vi "Keyence Handler_EP.vi"(8 "error in (no error)":errorcluster, 11 "Message Queues out":T5) -> (0 "error out":errorcluster, 3 "Message Queue":refnum<queue>)   [LabVIEW 2014]
uses:
  support/Message Queue/Message Queue.lvlib
  support/Message Queue/Lossy Enqueue Message (Single).vi
  <vilib>/ErrorRing/Error Ring.xnode
  <vilib>/ethernetip/ethernetip.lvlib
  <vilib>/Utility/error.llb/Error Cluster From Error Code.vi
  <vilib>/ethernetip/ethernetip.llb/ethernetip.ctl
  JXC Data Cluster_EP.ctl
  Control_EP.ctl
  Status_EP.ctl
  support/Message Queue/Message Cluster.ctl
  support/Message Queue/All Message Queues.ctl
panel:
  out "JXC Data Cluster":T1={"State Text"="", "Communication Opened"=FALSE, "Ethernet IP Session"="", "Status"={"BUSY"=FALSE, "SVRE"=FALSE, "SETON"=FALSE, "INP"=FALSE, "ESTOP"=FALSE, "ALARM"=FALSE, "READY"=FALSE, "Current Position"=0, "Current Position mm"=0.0, "Current Speed"=0, "Current Pushing Force"=0, "Target Position"=0, "Target Position mm"=0.0, "Alarm"=0, "Record number"=0}, "Control"={"Record number"=0, "HOLD"=FALSE, "SVON"=FALSE, "DRIVE"=FALSE, "RESET"=FALSE, "SETUP"=FALSE, "JOG-"=FALSE, "JOG+"=FALSE, "FLGTH"=FALSE}, "network path"="192.168.1.250"}
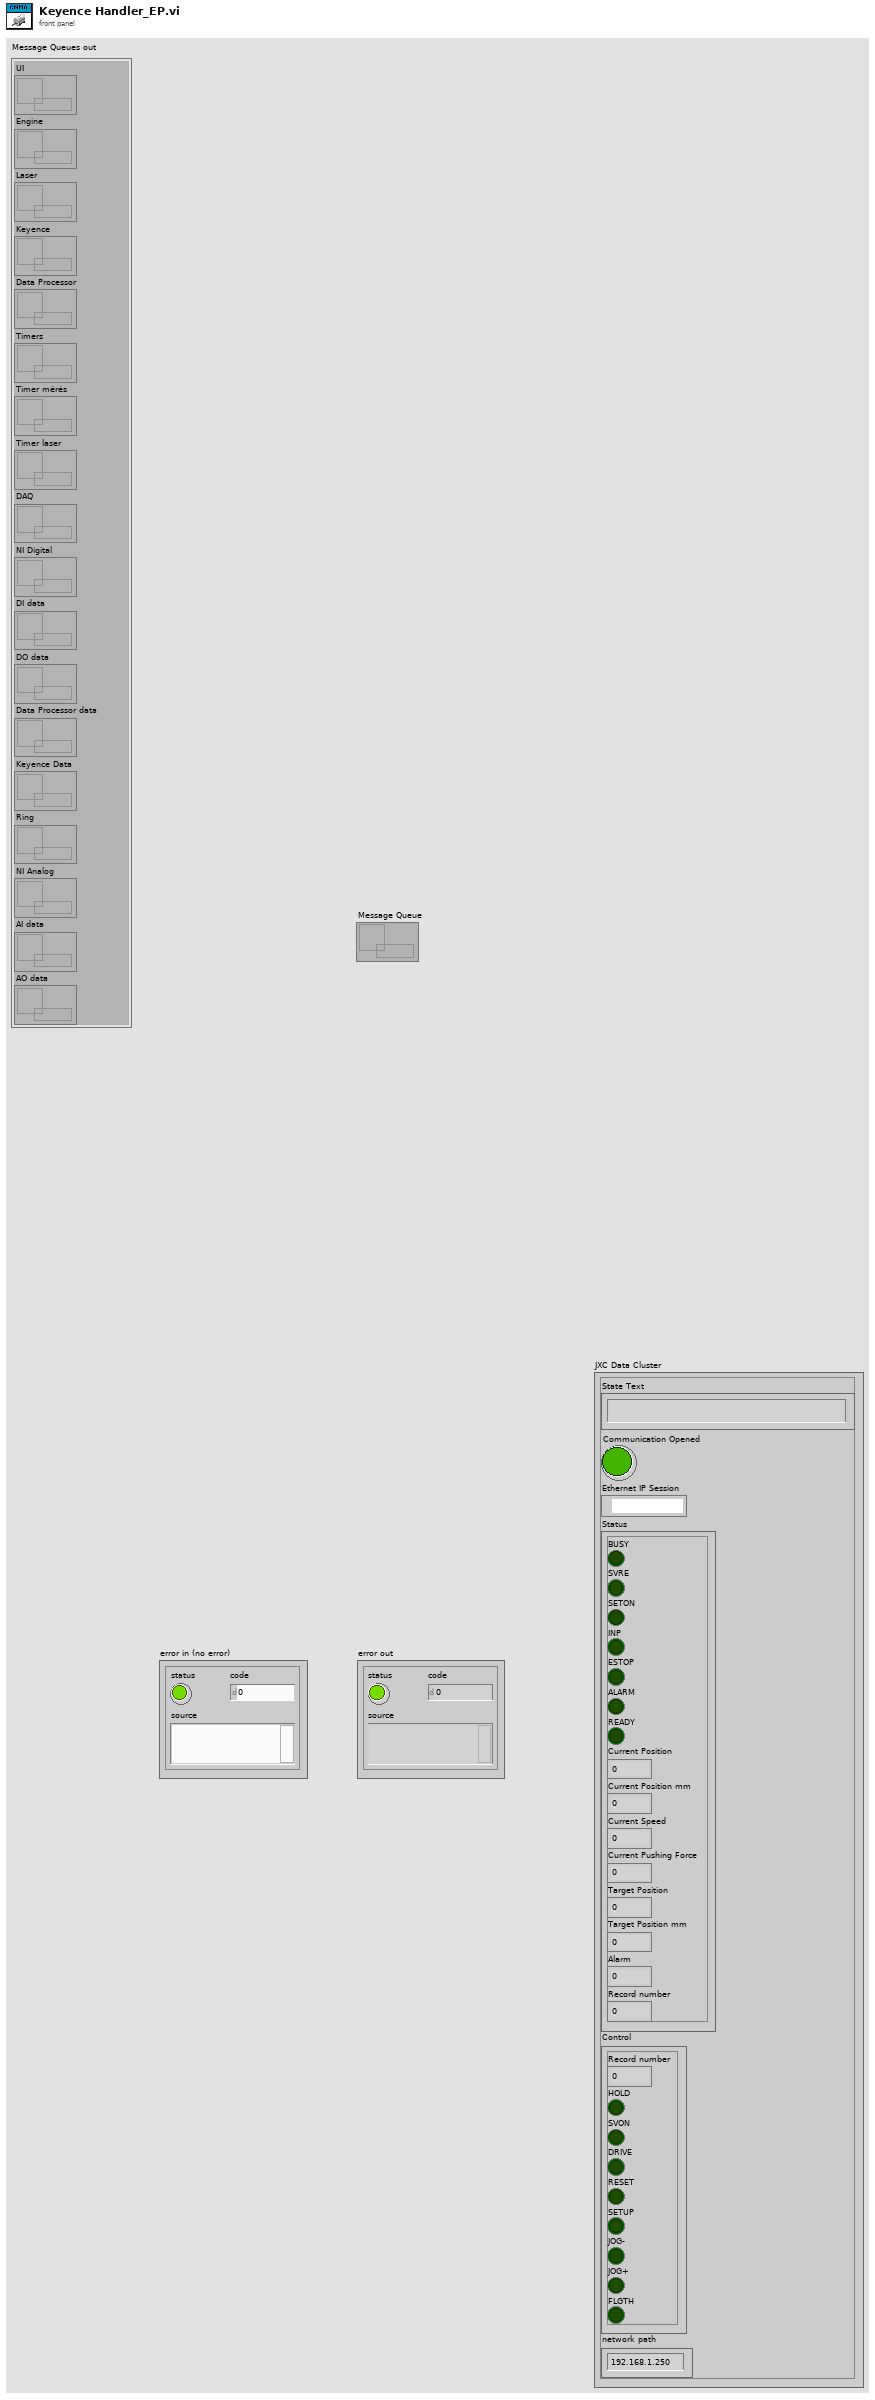
[diagram p1: front panel]
types:
  T1 = typedef "JXC Data Cluster_EP.ctl" = cluster{"State Text":string, "Communication Opened":bool, "Ethernet IP Session":T2, "Status":T3, "Control":T4, "network path":string}
  T2 = typedef "ethernetip.lvlib/ethernetip.ctl" = refnum<k21>
  T3 = typedef "Status_EP.ctl" = cluster{"BUSY":bool, "SVRE":bool, "SETON":bool, "INP":bool, "ESTOP":bool, "ALARM":bool, "READY":bool, "Current Position":u32, "Current Position mm":dbl, "Current Speed":u16, "Current Pushing Force":u16, "Target Position":u32, "Target Position mm":dbl, "Alarm":u8, "Record number":u32}
  T4 = typedef "Control_EP.ctl" = cluster{"Record number":u32, "HOLD":bool, "SVON":bool, "DRIVE":bool, "RESET":bool, "SETUP":bool, "JOG-":bool, "JOG+":bool, "FLGTH":bool}
  T5 = typedef "Message Queue.lvlib/All Message Queues.ctl" = cluster{"UI":refnum<queue>, "Engine":refnum<queue>, "Laser":refnum<queue>, "Keyence":refnum<queue>, "Data Processor":refnum<queue>, "Timers":refnum<queue>, "Timer mérés":refnum<queue>, "Timer laser":refnum<queue>, "DAQ":refnum<queue>, "NI Digital":refnum<queue>, "DI data":refnum<queue>, "DO data":refnum<queue>, "Data Processor data":refnum<queue>, "Keyence Data":refnum<queue>, "Ring":refnum<queue>, "NI Analog":refnum<queue>, "AI data":refnum<queue>, "AO data":refnum<queue>}
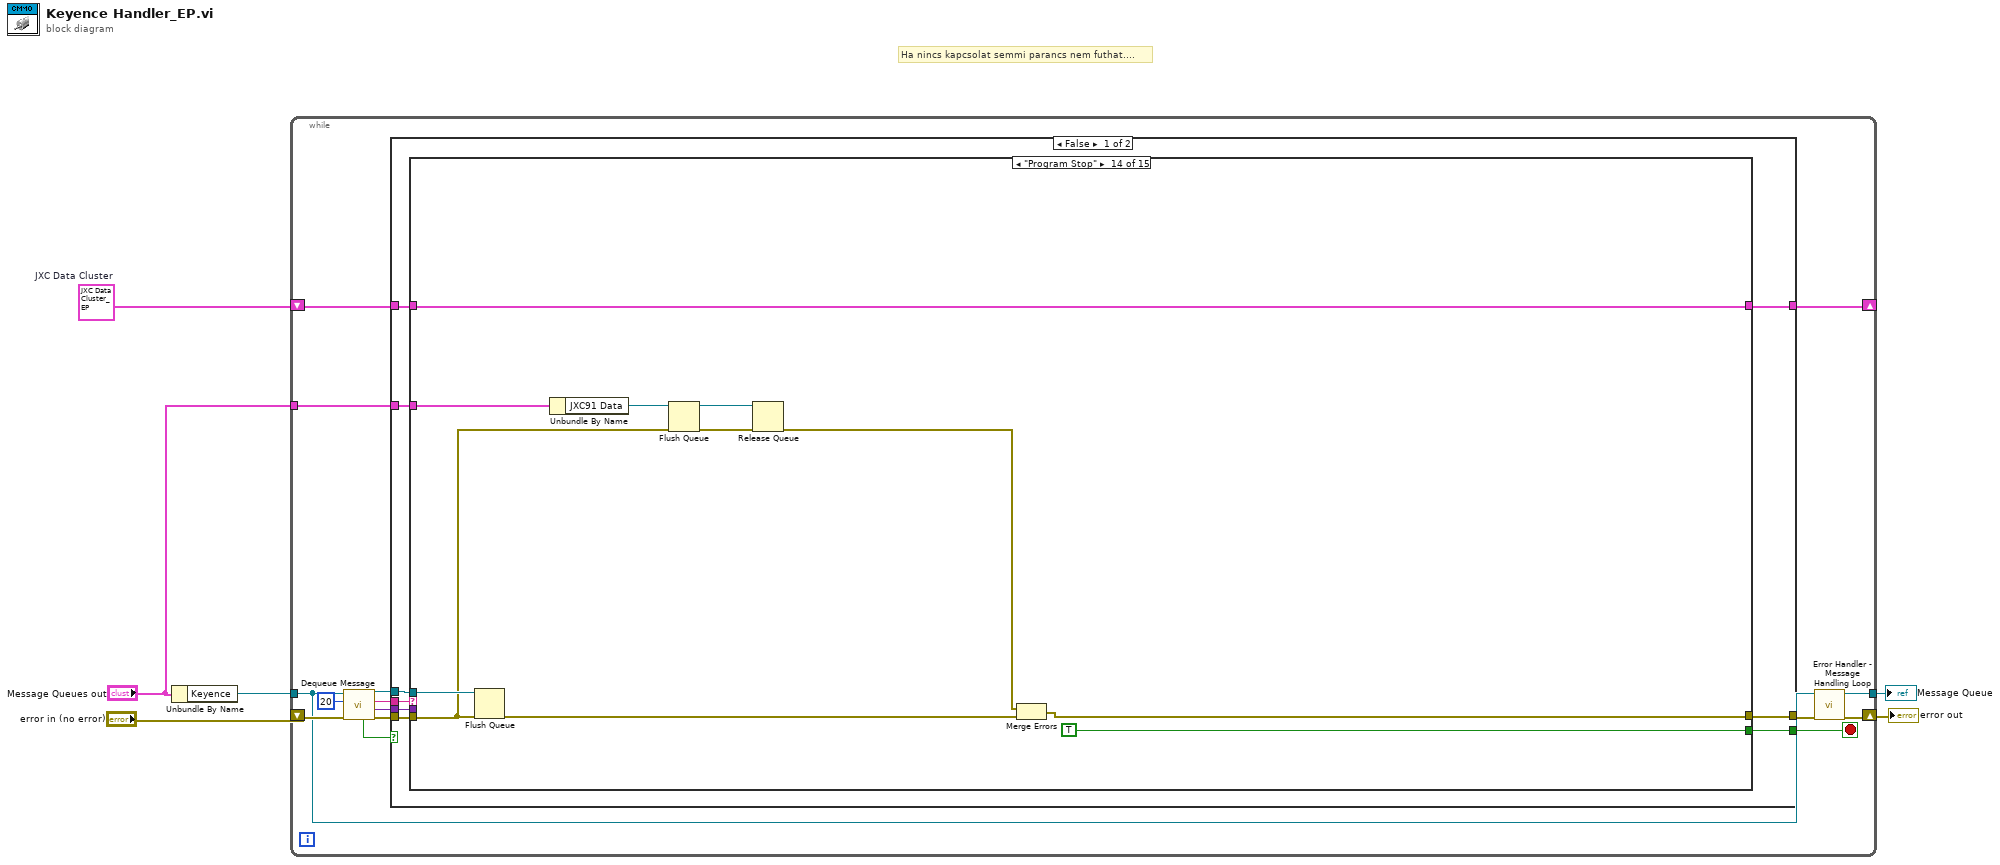
[diagram p0: block diagram]
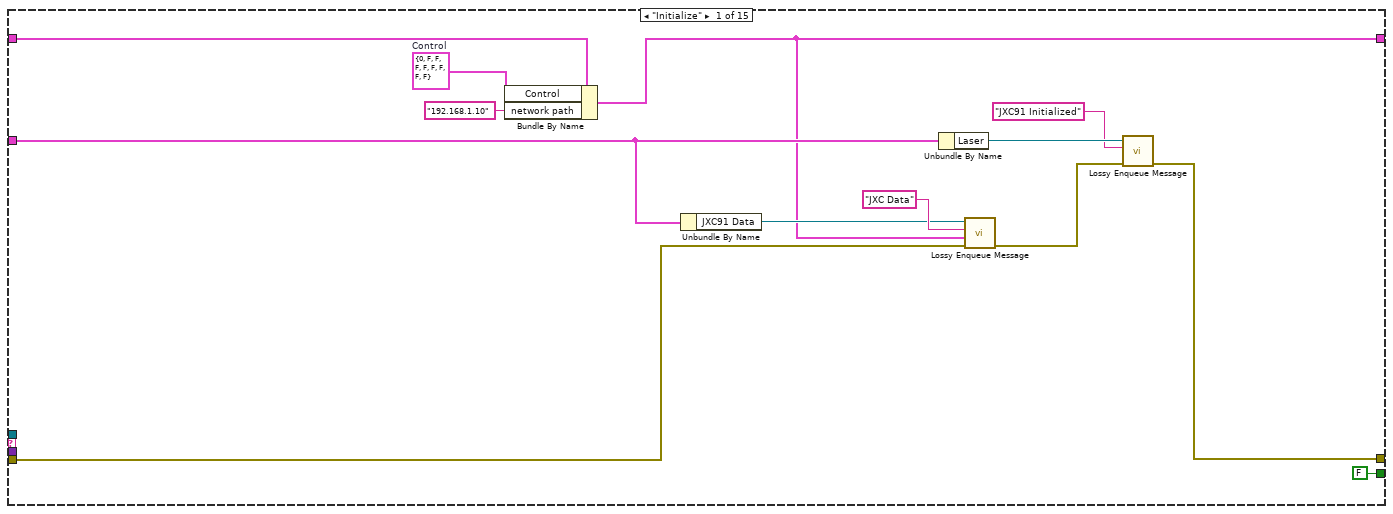
[diagram p2: hidden frame]
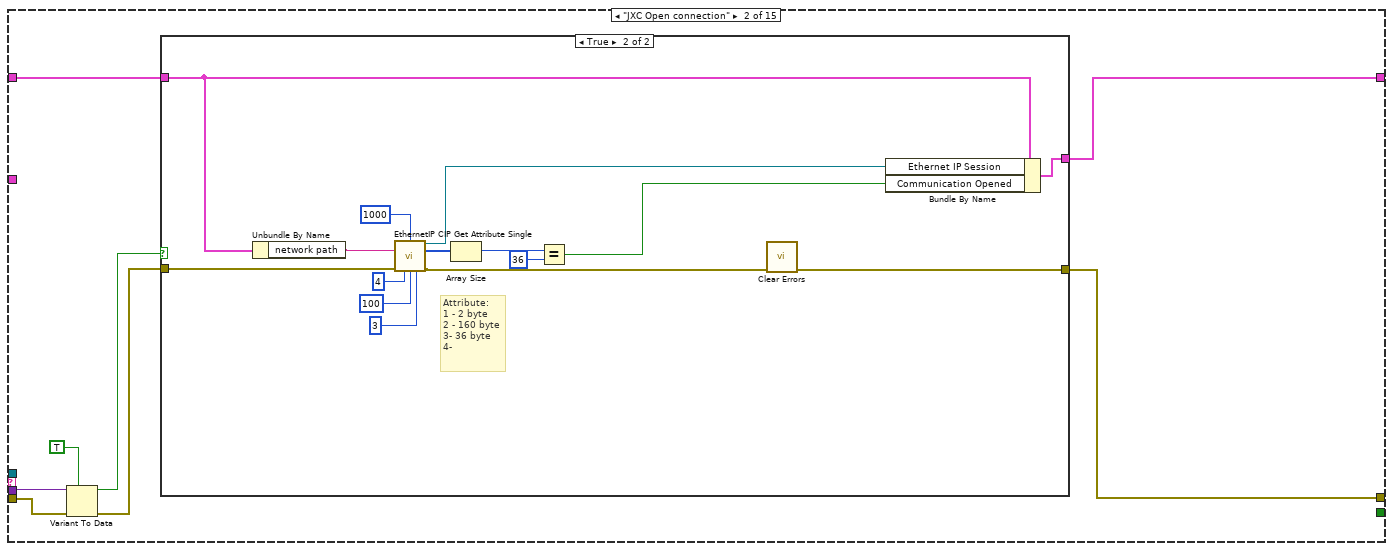
[diagram p3: hidden frame]
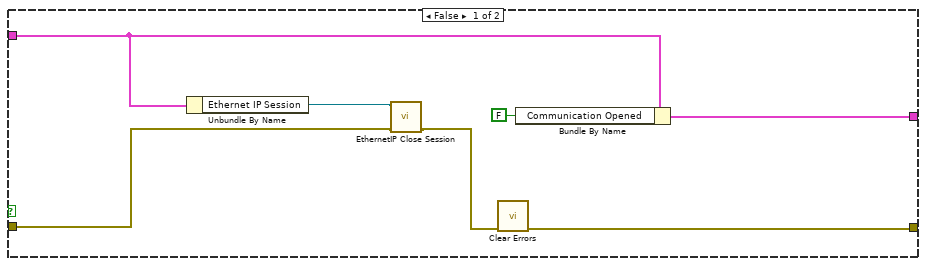
[diagram p4: hidden frame]
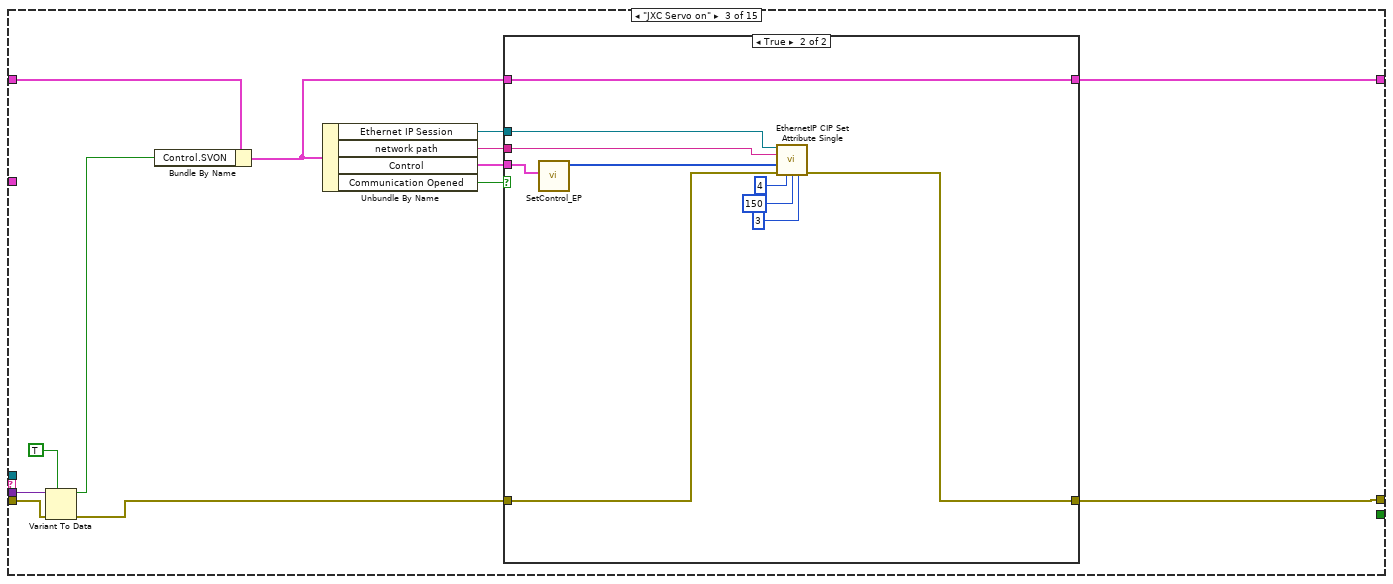
[diagram p5: hidden frame]
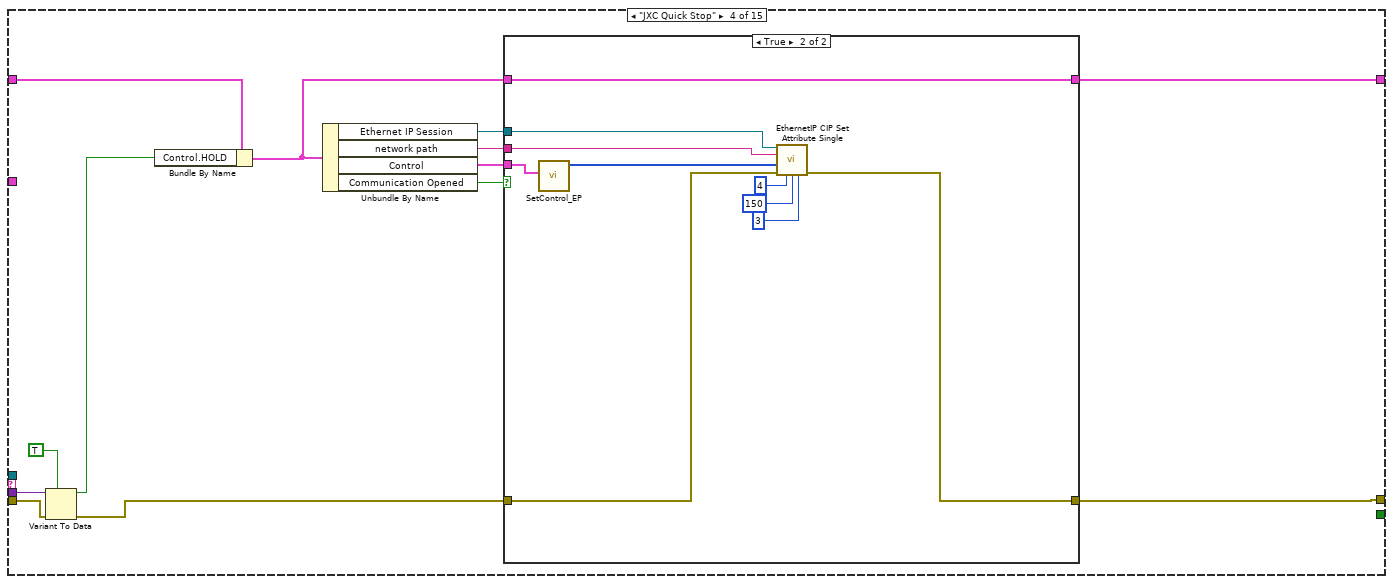
[diagram p7: hidden frame]
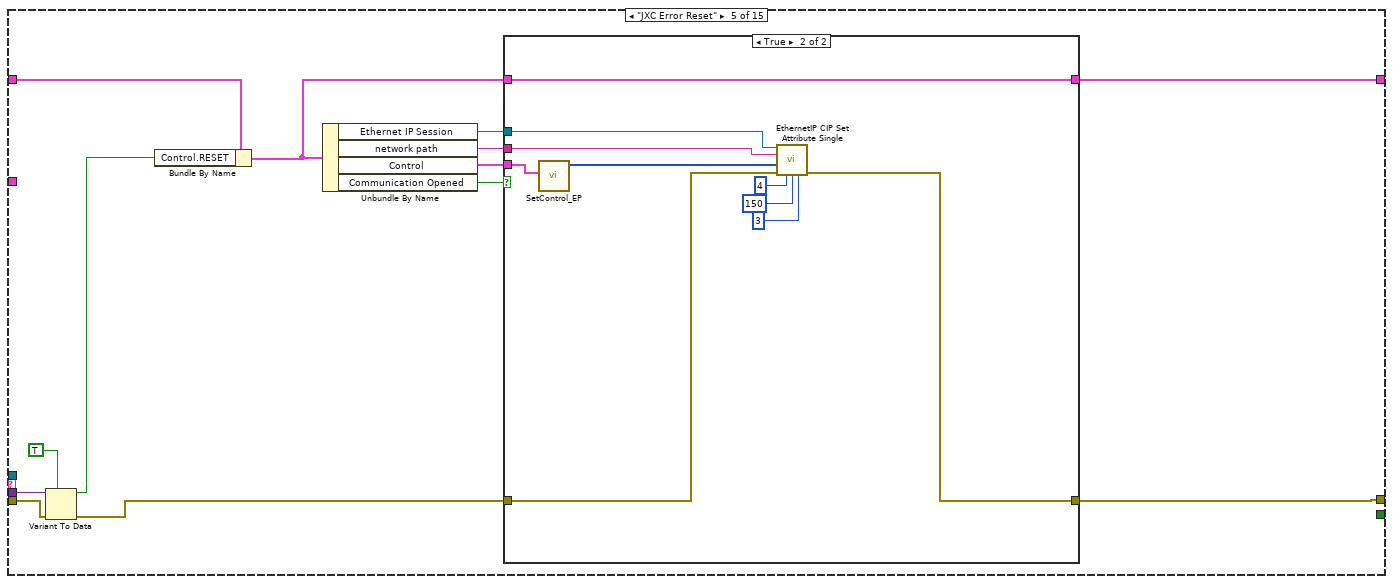
[diagram p9: hidden frame]
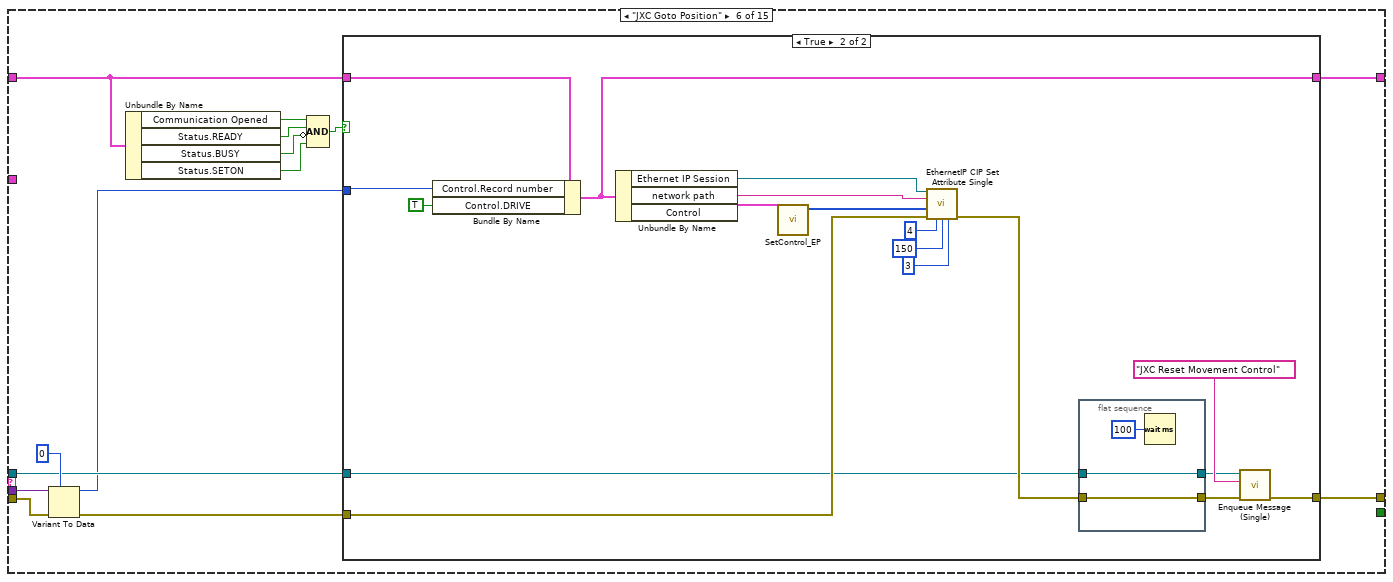
[diagram p11: hidden frame]
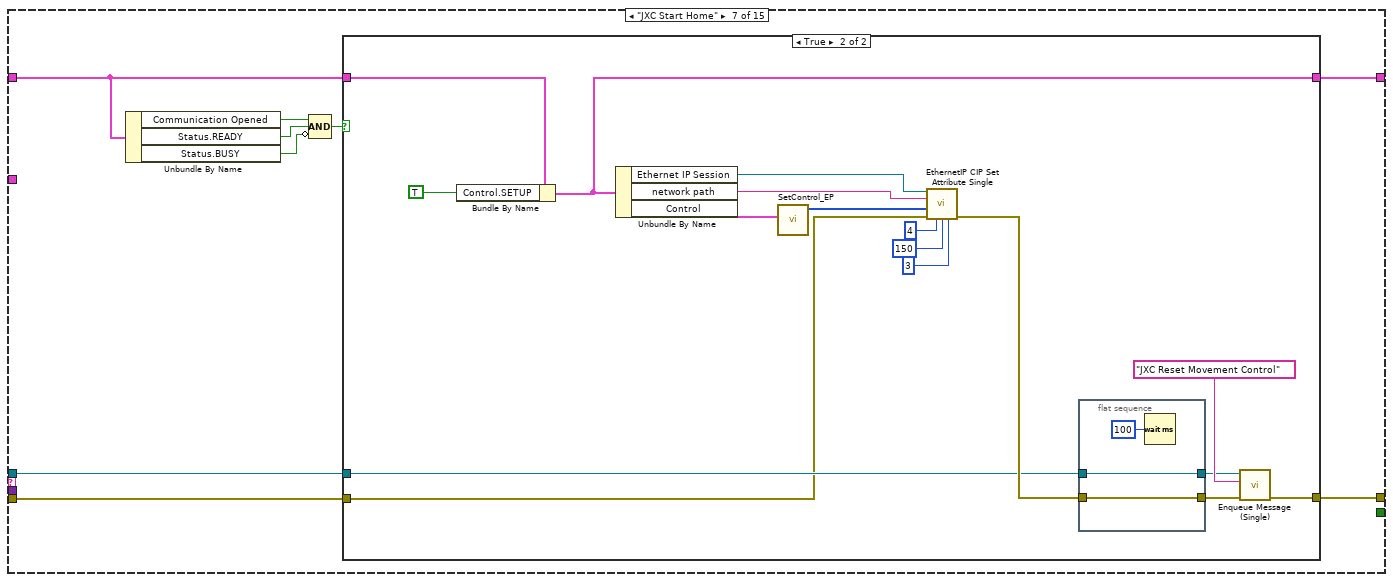
[diagram p13: hidden frame]
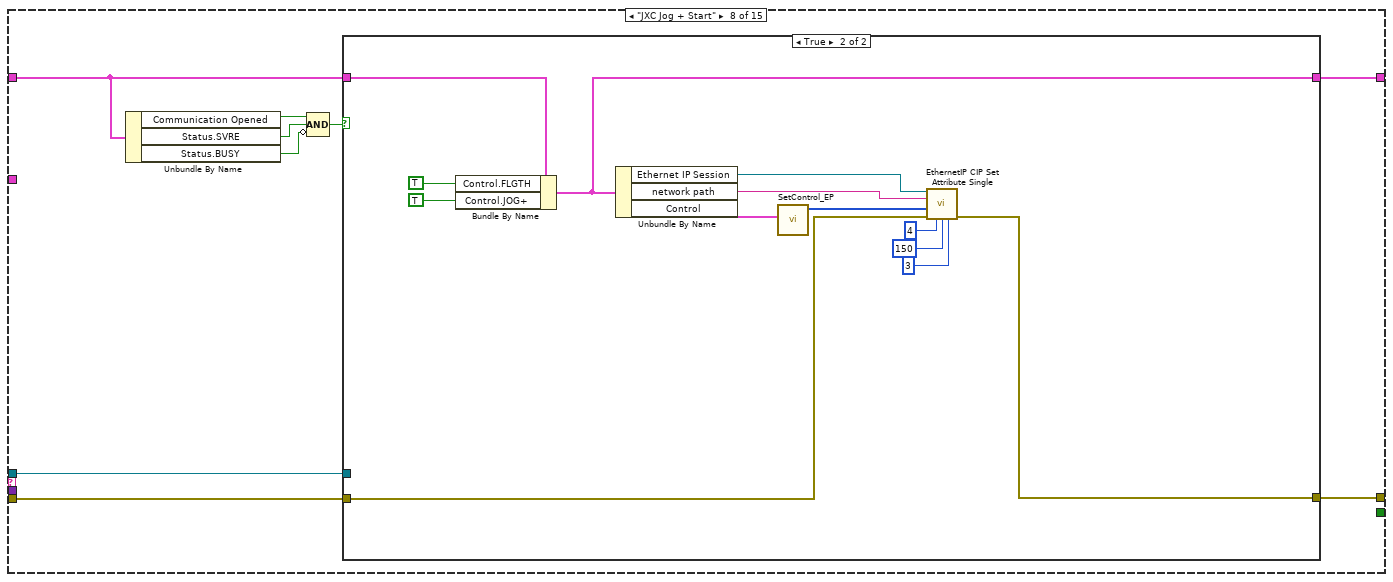
[diagram p15: hidden frame]
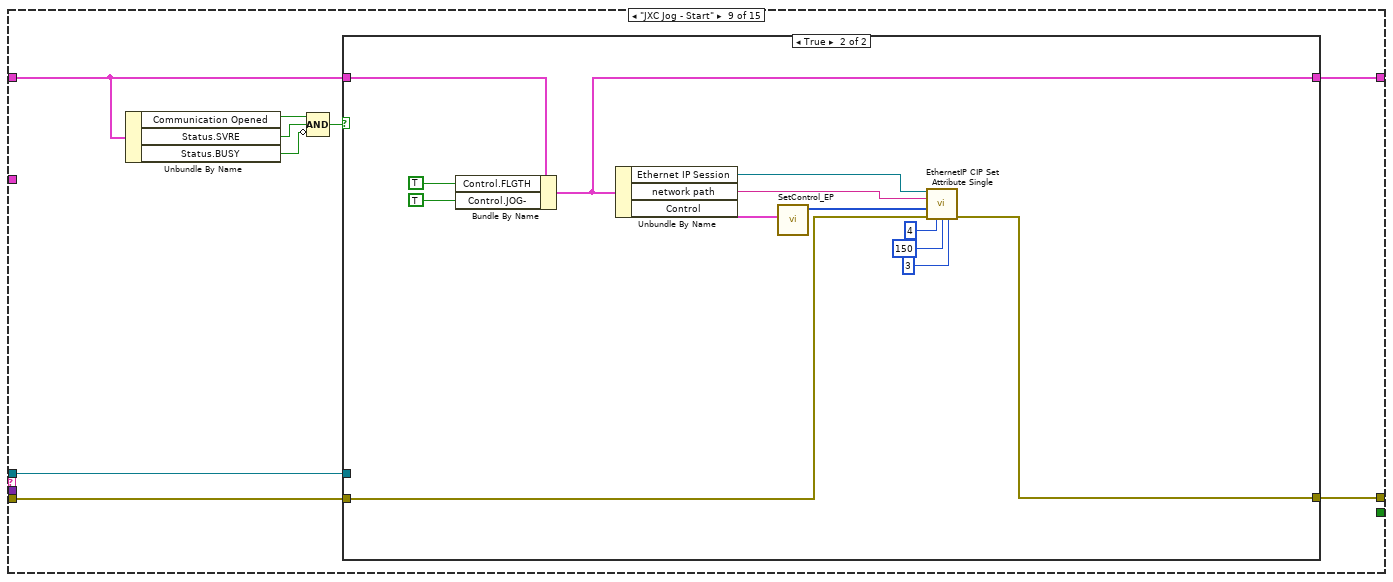
[diagram p17: hidden frame]
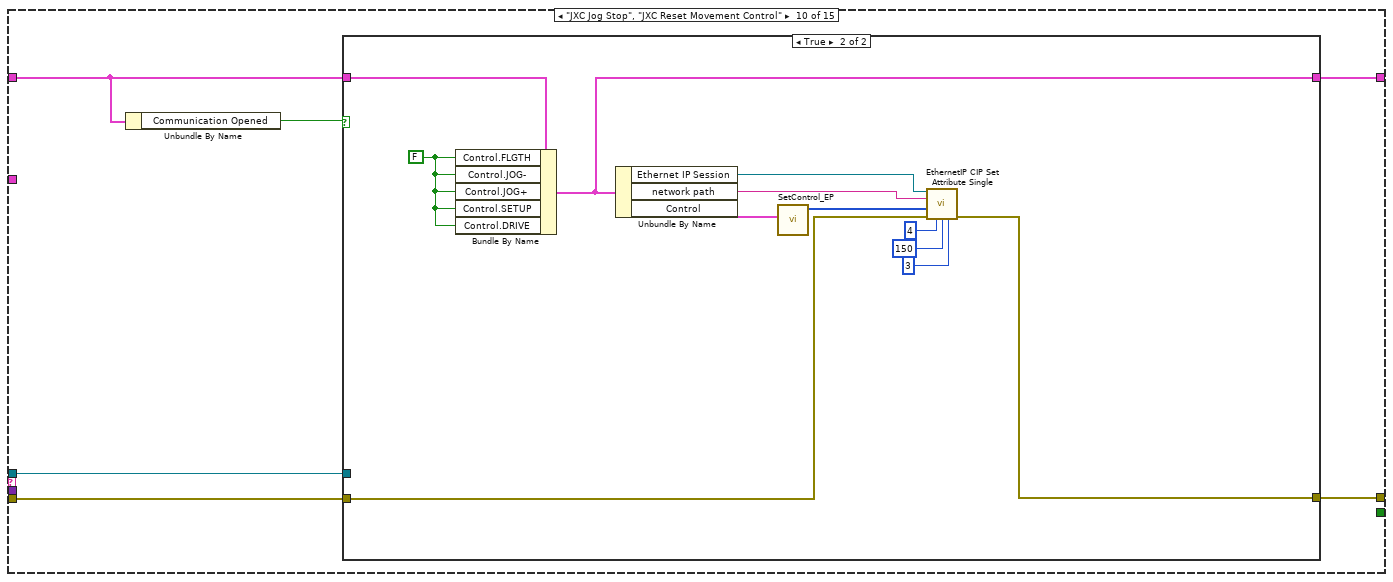
[diagram p19: hidden frame]
diagram:
  w1 = T1 {"State Text"="", "Communication Opened"=FALSE, "Ethernet IP Session"="", "Status"={"BUSY"=FALSE, "SVRE"=FALSE, "SETON"=FALSE, "INP"=FALSE, "ESTOP"=FALSE, "ALARM"=FALSE, "READY"=FALSE, "Current Position"=0, "Current Position mm"=0.0, "Current Speed"=0, "Current Pushing Force"=0, "Target Position"=0, "Target Position mm"=0.0, "Alarm"=0, "Record number"=0}, "Control"={"Record number"=0, "HOLD"=FALSE, "SVON"=FALSE, "DRIVE"=FALSE, "RESET"=FALSE, "SETUP"=FALSE, "JOG-"=FALSE, "JOG+"=FALSE, "FLGTH"=FALSE}, "network path"="*.*.*.*"}  # JXC Data Cluster
  # "Ha nincs kapcsolat semmi parancs nem futhat...."
  n1 = Unbundle By Name("Message Queues out") -> ("Keyence"=w3:refnum<queue>)
  n2 = while {
    tunnel: w3 -> [w10]
    shift-right: [w13] -> w6
    shift-left: "error in (no error)" -> [w21]
    tunnel: "Message Queues out" -> [w11]
    tunnel: [w9] -> w2
    shift-right: [w7] -> _
    shift-left: w1 -> [w8]
    stop <- w17 stop-if-true
    n3 = call "Dequeue Message.vi"("error in (no error)"=w21, "timeout in ms (-1)"=20, "Message Queue"=w10) -> ("error out"=w19:errorcluster, "Message Data"=w14:variant, "Message"=w20:string, "dup Message Queue"=w18:refnum<queue>, "timed out?"=w15:bool)  [unwired: 4 in]
    n4 = case shown="False" w15 {
      tunnel: w20 -> [w30 _]
      tunnel: w19 -> [w29 w343]
      tunnel: w18 -> [w28 _]
      tunnel: [w27 _] -> w17
      tunnel: [w26 w340] -> w12
      tunnel: w14 -> [w25 _]
      tunnel: w11 -> [w24 w342]
      tunnel: w8 -> [w23 w338]
      tunnel: [w22 w335] -> w7
      frame False {
        n5 = case shown="\"Program Stop\"" w30 {
          selector: w30 -> [_ _ _ _ _ _ _ _ _ _ _ _ _ _ w324]
          tunnel: w29 -> [w35 w46 w82 w107 w132 w160 w190 w221 w245 w266 w288 w289 w302 w316 _]
          tunnel: w28 -> [_ _ _ _ _ w157 w193 w224 w248 w269 w287 w298 w310 w323 _]
          tunnel: [w40 w49 w86 w111 w136 w156 w192 w223 w247 w268 w286 w294 w311 w313 w325] -> w26
          tunnel: [FALSE _ _ _ _ _ _ _ _ _ _ _ FALSE TRUE FALSE] -> w27
          tunnel: w25 -> [_ w47 w83 w108 w133 w161 _ _ _ _ _ w290 _ _ _]
          tunnel: w24 -> [w36 _ _ _ _ _ _ _ _ _ _ w297 _ w317 _]
          tunnel: w23 -> [w39 w51 w84 w109 w134 w155 w191 w222 w246 w267 w285 w292 w304 w321 w326]
          tunnel: [w33 w50 w85 w110 w135 w162 w194 w225 w249 w270 w285 w292 w303 w321 w326] -> w22
          frame "Initialize" {
            w32 = T4 {"Record number"=0, "HOLD"=FALSE, "SVON"=FALSE, "DRIVE"=FALSE, "RESET"=FALSE, "SETUP"=FALSE, "JOG-"=FALSE, "JOG+"=FALSE, "FLGTH"=FALSE}  # Control
            n6 = Bundle By Name(cluster=w39, "Control"=w32, "network path"="192.168.1.10") -> (w33:T1)
            n7 = Unbundle By Name(w36) -> ("JXC91 Data"=w37:refnum<queue>)
            n8 = Unbundle By Name(w36) -> ("Laser"=w42:refnum<queue>)
            n9 = call-poly "Lossy Enqueue Message.vi"("error in (no error)"=w35, "Message Data"=w33, "Message"="JXC Data", "Message Queue"=w37) -> ("error out"=w34:errorcluster)  [unwired: 6 in, 1 out]
            n10 = call-poly "Lossy Enqueue Message.vi"("error in (no error)"=w34, "Message"="JXC91 Initialized", "Message Queue"=w42) -> ("error out"=w40:errorcluster)  [unwired: 7 in, 1 out]
          }
          frame "JXC Open connection" {
            n11 = Variant To Data(error in=w46, type=TRUE ("Control word.Enable Voltage"), Variant=w47) -> (data=w44:bool, error out=w45:errorcluster)
            n12 = case shown="True" w44 {
              tunnel: w45 -> [w54 w71]
              tunnel: w51 -> [w57 w60]
              tunnel: [w58 w73] -> w50
              tunnel: [w55 w72] -> w49
              frame False {
                n13 = Unbundle By Name(w57) -> ("Ethernet IP Session"=w52:T2)
                n14 = call <vilib>:"EthernetIP Close Session.vi"("error in"=w54, "Session in"=w52) -> ("error out"=w53:errorcluster)  [unwired: 9 in]
                n15 = call <vilib>:"Clear Errors.vi"("error in (no error)"=w53) -> ("error out"=w55:errorcluster)  [unwired: 5 in, 1 out]
                n16 = Bundle By Name(cluster=w57, "Communication Opened"=FALSE) -> (w58:T1)
              }
              frame True {
                # "Attribute: \n1 - 2 byte\n2 - 160 byte\n3- 36 byte\n4-"
                n17 = Unbundle By Name(w60) -> ("network path"=w59:string)
                n18 = call <vilib>:"EthernetIP CIP Get Attribute Single.vi"("Timeout (ms)"=1000, "Network Path"=w59, "error in"=w71, "Class"=4, "Instance"=u32 100, "Attribute"=3) -> ("Session out"=w69:T2, "Data"=w64:u8[], "error out"=w70:errorcluster)  [unwired: 7 in]
                n19 = Array Size(array=w64) -> (size(s)=w63:i32)
                n20 = Equal?(x=w63, y=36) -> (x = y?=w61:bool)
                n21 = call <vilib>:"Clear Errors.vi"("error in (no error)"=w70) -> ("error out"=w72:errorcluster)  [unwired: 5 in, 1 out]
                n22 = Bundle By Name(cluster=w60, "Ethernet IP Session"=w69, "Communication Opened"=w61) -> (w73:T1)
              }
            }
          }
          frame "JXC Servo on" {
            n23 = Variant To Data(error in=w82, type=TRUE ("Control word.Enable Voltage"), Variant=w83) -> (data=w79:bool, error out=w81:errorcluster)
            n24 = Bundle By Name(cluster=w84, "Control.SVON"=w79) -> (w78:T1)
            n25 = Unbundle By Name(w78) -> ("Ethernet IP Session"=w75:T2, "network path"=w74:string, "Control"=w76:T4, "Communication Opened"=w77:bool)
            n26 = case shown="True" w77 {
              tunnel: [w87 w97] -> w86
              tunnel: [w88 w93] -> w85
              tunnel: w81 -> [w87 w98]
              tunnel: w78 -> [w88 w93]
              tunnel: w76 -> [_ w92]
              tunnel: w75 -> [_ w89]
              tunnel: w74 -> [_ w90]
              frame False {
              }
              frame True {
                n27 = call "SetControl_EP.vi"(10:w92) -> ("Data"=w91:u8[])  [unwired: 10 in]
                n28 = call <vilib>:"EthernetIP CIP Set Attribute Single.vi"("Session in"=w89, "Network Path"=w90, "Data"=w91, "error in"=w98, "Class"=4, "Instance"=u32 150, "Attribute"=3) -> ("error out"=w97:errorcluster)  [unwired: 7 in, 1 out]
              }
            }
          }
          frame "JXC Quick Stop" {
            n29 = Variant To Data(error in=w107, type=TRUE ("Control word.Enable Voltage"), Variant=w108) -> (data=w104:bool, error out=w106:errorcluster)
            n30 = Bundle By Name(cluster=w109, "Control.HOLD"=w104) -> (w103:T1)
            n31 = Unbundle By Name(w103) -> ("Ethernet IP Session"=w100:T2, "network path"=w99:string, "Control"=w101:T4, "Communication Opened"=w102:bool)
            n32 = case shown="True" w102 {
              tunnel: [w112 w122] -> w111
              tunnel: [w113 w118] -> w110
              tunnel: w106 -> [w112 w123]
              tunnel: w103 -> [w113 w118]
              tunnel: w101 -> [_ w117]
              tunnel: w100 -> [_ w114]
              tunnel: w99 -> [_ w115]
              frame False {
              }
              frame True {
                n33 = call "SetControl_EP.vi"(10:w117) -> ("Data"=w116:u8[])  [unwired: 10 in]
                n34 = call <vilib>:"EthernetIP CIP Set Attribute Single.vi"("Session in"=w114, "Network Path"=w115, "Data"=w116, "error in"=w123, "Class"=4, "Instance"=u32 150, "Attribute"=3) -> ("error out"=w122:errorcluster)  [unwired: 7 in, 1 out]
              }
            }
          }
          frame "JXC Error Reset" {
            n35 = Variant To Data(error in=w132, type=TRUE ("Control word.Enable Voltage"), Variant=w133) -> (data=w129:bool, error out=w131:errorcluster)
            n36 = Bundle By Name(cluster=w134, "Control.RESET"=w129) -> (w128:T1)
            n37 = Unbundle By Name(w128) -> ("Ethernet IP Session"=w125:T2, "network path"=w124:string, "Control"=w126:T4, "Communication Opened"=w127:bool)
            n38 = case shown="True" w127 {
              tunnel: [w137 w147] -> w136
              tunnel: [w138 w143] -> w135
              tunnel: w131 -> [w137 w148]
              tunnel: w128 -> [w138 w143]
              tunnel: w126 -> [_ w142]
              tunnel: w125 -> [_ w139]
              tunnel: w124 -> [_ w140]
              frame False {
              }
              frame True {
                n39 = call "SetControl_EP.vi"(10:w142) -> ("Data"=w141:u8[])  [unwired: 10 in]
                n40 = call <vilib>:"EthernetIP CIP Set Attribute Single.vi"("Session in"=w139, "Network Path"=w140, "Data"=w141, "error in"=w148, "Class"=4, "Instance"=u32 150, "Attribute"=3) -> ("error out"=w147:errorcluster)  [unwired: 7 in, 1 out]
              }
            }
          }
          frame "JXC Goto Position" {
            n41 = Variant To Data(error in=w160, type=u8 0 ("Record number"), Variant=w161) -> (data=w154:u8, error out=w158:errorcluster)
            n42 = Unbundle By Name(w155) -> ("Communication Opened"=w152:bool, "Status.READY"=w151:bool, "Status.BUSY"=w150:bool, "Status.SETON"=w149:bool)
            n43 = Compound Arithmetic op=AND(w152, w151, invert w150, w149) -> (w153:bool)
            n44 = case shown="True" w153 {
              tunnel: [w164 w173] -> w162
              tunnel: w158 -> [w163 w171]
              tunnel: w157 -> [_ w167]
              tunnel: [w163 w182] -> w156
              tunnel: w155 -> [w164 w180]
              tunnel: w154 -> [_ w179]
              frame False {
              }
              frame True {
                n45 = Bundle By Name(cluster=w180, "Control.Record number"=w179, "Control.DRIVE"=TRUE) -> (w173:T1)
                n46 = Unbundle By Name(w173) -> ("Ethernet IP Session"=w166:T2, "network path"=w165:string, "Control"=w172:T4)
                n47 = call "SetControl_EP.vi"(10:w172) -> ("Data"=w174:u8[])  [unwired: 10 in]
                n48 = call <vilib>:"EthernetIP CIP Set Attribute Single.vi"("Session in"=w166, "Network Path"=w165, "Data"=w174, "error in"=w171, "Class"=4, "Instance"=u32 150, "Attribute"=3) -> ("error out"=w170:errorcluster)  [unwired: 7 in, 1 out]
                n49 = flat-sequence {
                  tunnel: [w184] -> w169
                  tunnel: w170 -> [w184]
                  tunnel: [w183] -> w168
                  tunnel: w167 -> [w183]
                  frame #0 {
                    n50 = Wait (ms)(milliseconds to wait=u32 100) -> ()  [unwired: 1 out]
                  }
                }
                n51 = call "Enqueue Message (Single).vi"("error in (no error)"=w169, "Message"="JXC Reset Movement Control", "Message Queue"=w168) -> ("error out"=w182:errorcluster)  [unwired: 7 in, 1 out]
              }
            }
          }
          frame "JXC Start Home" {
            n52 = Unbundle By Name(w191) -> ("Communication Opened"=w189:bool, "Status.READY"=w188:bool, "Status.BUSY"=w187:bool)
            n53 = Compound Arithmetic op=AND(w189, w188, invert w187) -> (w186:bool)
            n54 = case shown="True" w186 {
              tunnel: [w196 w205] -> w194
              tunnel: w193 -> [_ w200]
              tunnel: [w195 w213] -> w192
              tunnel: w191 -> [w196 w211]
              tunnel: w190 -> [w195 w199]
              frame False {
              }
              frame True {
                n55 = Bundle By Name(cluster=w211, "Control.SETUP"=TRUE ("Control.DRIVE")) -> (w205:T1)
                n56 = Unbundle By Name(w205) -> ("Ethernet IP Session"=w198:T2, "network path"=w197:string, "Control"=w204:T4)
                n57 = call "SetControl_EP.vi"(10:w204) -> ("Data"=w206:u8[])  [unwired: 10 in]
                n58 = call <vilib>:"EthernetIP CIP Set Attribute Single.vi"("Session in"=w198, "Network Path"=w197, "Data"=w206, "error in"=w199, "Class"=4, "Instance"=u32 150, "Attribute"=3) -> ("error out"=w203:errorcluster)  [unwired: 7 in, 1 out]
                n59 = flat-sequence {
                  tunnel: [w215] -> w202
                  tunnel: w203 -> [w215]
                  tunnel: [w214] -> w201
                  tunnel: w200 -> [w214]
                  frame #0 {
                    n60 = Wait (ms)(milliseconds to wait=u32 100) -> ()  [unwired: 1 out]
                  }
                }
                n61 = call "Enqueue Message (Single).vi"("error in (no error)"=w202, "Message"="JXC Reset Movement Control", "Message Queue"=w201) -> ("error out"=w213:errorcluster)  [unwired: 7 in, 1 out]
              }
            }
          }
          frame "JXC Jog + Start" {
            n62 = Unbundle By Name(w222) -> ("Communication Opened"=w220:bool, "Status.SVRE"=w219:bool, "Status.BUSY"=w218:bool)
            n63 = Compound Arithmetic op=AND(w220, w219, invert w218) -> (w217:bool)
            n64 = case shown="True" w217 {
              tunnel: [w227 w234] -> w225
              tunnel: w224 -> [_ _]
              tunnel: [w226 w231] -> w223
              tunnel: w222 -> [w227 w240]
              tunnel: w221 -> [w226 w230]
              frame False {
              }
              frame True {
                n65 = Bundle By Name(cluster=w240, "Control.FLGTH"=TRUE ("Control.DRIVE"), "Control.JOG+"=TRUE) -> (w234:T1)
                n66 = Unbundle By Name(w234) -> ("Ethernet IP Session"=w229:T2, "network path"=w228:string, "Control"=w233:T4)
                n67 = call "SetControl_EP.vi"(10:w233) -> ("Data"=w235:u8[])  [unwired: 10 in]
                n68 = call <vilib>:"EthernetIP CIP Set Attribute Single.vi"("Session in"=w229, "Network Path"=w228, "Data"=w235, "error in"=w230, "Class"=4, "Instance"=u32 150, "Attribute"=3) -> ("error out"=w231:errorcluster)  [unwired: 7 in, 1 out]
              }
            }
          }
          frame "JXC Jog - Start" {
            n69 = Unbundle By Name(w246) -> ("Communication Opened"=w244:bool, "Status.SVRE"=w243:bool, "Status.BUSY"=w242:bool)
            n70 = Compound Arithmetic op=AND(w244, w243, invert w242) -> (w241:bool)
            n71 = case shown="True" w241 {
              tunnel: [w251 w258] -> w249
              tunnel: w248 -> [_ _]
              tunnel: [w250 w255] -> w247
              tunnel: w246 -> [w251 w264]
              tunnel: w245 -> [w250 w254]
              frame False {
              }
              frame True {
                n72 = Bundle By Name(cluster=w264, "Control.FLGTH"=TRUE ("Control.DRIVE"), "Control.JOG-"=TRUE ("Control.JOG+")) -> (w258:T1)
                n73 = Unbundle By Name(w258) -> ("Ethernet IP Session"=w253:T2, "network path"=w252:string, "Control"=w257:T4)
                n74 = call "SetControl_EP.vi"(10:w257) -> ("Data"=w259:u8[])  [unwired: 10 in]
                n75 = call <vilib>:"EthernetIP CIP Set Attribute Single.vi"("Session in"=w253, "Network Path"=w252, "Data"=w259, "error in"=w254, "Class"=4, "Instance"=u32 150, "Attribute"=3) -> ("error out"=w255:errorcluster)  [unwired: 7 in, 1 out]
              }
            }
          }
          frame "JXC Jog Stop", "JXC Reset Movement Control" {
            n76 = Unbundle By Name(w267) -> ("Communication Opened"=w265:bool)
            n77 = case shown="True" w265 {
              tunnel: [w272 w279] -> w270
              tunnel: w269 -> [_ _]
              tunnel: [w271 w277] -> w268
              tunnel: w267 -> [w272 w284]
              tunnel: w266 -> [w271 w276]
              frame False {
              }
              frame True {
                w275 = FALSE ("Control.DRIVE")
                n78 = Bundle By Name(cluster=w284, "Control.FLGTH"=w275, "Control.JOG-"=w275, "Control.JOG+"=w275, "Control.SETUP"=w275, "Control.DRIVE"=w275) -> (w279:T1)
                n79 = Unbundle By Name(w279) -> ("Ethernet IP Session"=w274:T2, "network path"=w273:string, "Control"=w278:T4)
                n80 = call "SetControl_EP.vi"(10:w278) -> ("Data"=w280:u8[])  [unwired: 10 in]
                n81 = call <vilib>:"EthernetIP CIP Set Attribute Single.vi"("Session in"=w274, "Network Path"=w273, "Data"=w280, "error in"=w276, "Class"=4, "Instance"=u32 150, "Attribute"=3) -> ("error out"=w277:errorcluster)  [unwired: 7 in, 1 out]
              }
            }
          }
          frame "Abort" {
            n82 = Flush Queue(queue=w287, error in (no error)=w288) -> (error out=w286:errorcluster)  [unwired: 2 out]
          }
          frame "Error" {
            n83 = Unbundle By Name(w297) -> ("UI"=w296:refnum<queue>)
            n84 = call-poly "Enqueue Message.vi"("error in (no error)"=w289, "Message Data"=w290, "Message"="Error", "Message Queue"=w296) -> ("error out"=w293:errorcluster)  [unwired: 6 in, 1 out]
            n85 = call-poly "Enqueue Message.vi"("Priority Message? (F)"=TRUE, "error in (no error)"=w289, "Message"="Initiate Stop", "Message Queue"=w298) -> ("error out"=w295:errorcluster)  [unwired: 6 in, 1 out]
            n86 = Merge Errors(w293, w295) -> (w294:errorcluster)
          }
          frame "Initiate Stop" {
            n87 = Unbundle By Name(w304) -> ("Ethernet IP Session"=w305:T2)
            n88 = call <vilib>:"EthernetIP Close Session.vi"("error in"=w302, "Session in"=w305) -> ("error out"=w306:errorcluster)  [unwired: 9 in]
            n89 = call <vilib>:"Clear Errors.vi"("error in (no error)"=w306) -> ("error out"=w301:errorcluster)  [unwired: 5 in, 1 out]
            n90 = Bundle By Name(cluster=w304, "Communication Opened"=FALSE) -> (w303:T1)
            n91 = call-poly "Enqueue Message.vi"("Priority Message? (F)"=TRUE, "error in (no error)"=w301, "Message"="Program Stop", "Message Queue"=w310) -> ("error out"=w311:errorcluster)  [unwired: 6 in, 1 out]
          }
          frame "Program Stop" {
            n92 = Flush Queue(queue=w323, error in (no error)=w316) -> (error out=w315:errorcluster)  [unwired: 2 out]
            n93 = Unbundle By Name(w317) -> ("JXC91 Data"=w320:refnum<queue>)
            n94 = Flush Queue(queue=w320, error in (no error)=w316) -> (queue out=w319:refnum<queue>, error out=w318:errorcluster)  [unwired: 1 out]
            n95 = Release Queue(queue=w319, error in (no error)=w318) -> (error out=w314:errorcluster)  [unwired: 1 in, 2 out]
            n96 = Merge Errors(w314, w315) -> (w313:errorcluster)
          }
          frame Default {
            n97 = xnode "Error Ring"("parameter 0"=w324) -> ("error out"=w325:errorcluster)
          }
        }
      }
      frame True {
        n98 = Unbundle By Name(w338) -> ("Communication Opened"=w339:bool, "Ethernet IP Session"=w337:T2, "network path"=w336:string)
        n99 = Unbundle By Name(w342) -> ("JXC91 Data"=w341:refnum<queue>)
        n100 = case shown="True" w339 {
          tunnel: w343 -> [w346 w353]
          tunnel: w338 -> [w344 w360]
          tunnel: w341 -> [w345 w359]
          tunnel: [w347 w362] -> w340
          tunnel: [w344 w361] -> w335
          tunnel: w337 -> [_ w357]
          tunnel: w336 -> [_ w349]
          frame False {
            n101 = call-poly "Lossy Enqueue Message.vi"("error in (no error)"=w346, "Message Data"=w344, "Message"="JXC Data", "Message Queue"=w345) -> ("error out"=w347:errorcluster)  [unwired: 6 in, 1 out]
          }
          frame True {
            # "Attribute: \n1 - 2 byte\n2 - 160 byte\n3- 36 byte\n4-"
            n102 = call <vilib>:"EthernetIP CIP Get Attribute Single.vi"("Session in"=w357, "Timeout (ms)"=1000, "Network Path"=w349, "error in"=w353, "Class"=4, "Instance"=u32 100, "Attribute"=3) -> ("Data"=w351:u8[], "error out"=w350:errorcluster)  [unwired: 6 in, 1 out]
            n103 = call "GetStatus_EP.vi"("Data"=w351) -> ("Status"=w352:T3)  [unwired: 10 in]
            n104 = Bundle By Name(cluster=w360, "Status"=w352) -> (w361:T1)
            n105 = call-poly "Lossy Enqueue Message.vi"("error in (no error)"=w350, "Message Data"=w361, "Message"="JXC Data", "Message Queue"=w359) -> ("error out"=w362:errorcluster)  [unwired: 6 in, 1 out]
          }
        }
        "JXC Data Cluster" <- w335
      }
    }
    n106 = call "Error Handler - Message Handling Loop.vi"("error in (no error)"=w12, "Message Queue"=w10) -> ("dup error in"=w13:errorcluster, "dup Message Queue"=w9:refnum<queue>)  [unwired: 8 in]
  }
  "error out" <- w6
  "Message Queue" <- w2
